vi "SetText.vi"(4 "Alignment":T1, 5 "Alpha":dbl=1.0, 7 "Color":u32(colorbox), 8 "error in (no error)":errorcluster, 9 "Font Path":path, 10 "Text":string, 11 "3D Object in":refnum<class "3D Object.lvclass">) -> (0 "error out":errorcluster, 3 "3D Object out":refnum<class "3D Object.lvclass">)   [LabVIEW 2015, in "3D Object.lvclass"]
uses:
  3D Object.lvclass
  <vilib>/Utility/miscctls.llb/LVSceneTextAlignment.ctl
  3D Object.lvclass/3D Object.ctl
  <vilib>/picture/3D Picture Control/NI_3D Picture Control.lvlib
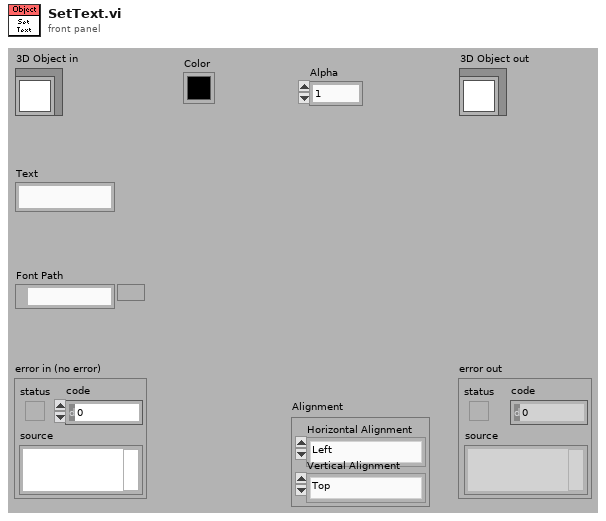
[diagram p1: front panel]
types:
  T1 = typedef "LVSceneTextAlignment.ctl" = cluster{"Horizontal Alignment":enum8{"Left", "Right", "Center"}, "Vertical Alignment":enum8{"Top", "Bottom", "Center", "Base Line", "Bottom Base Line"}}
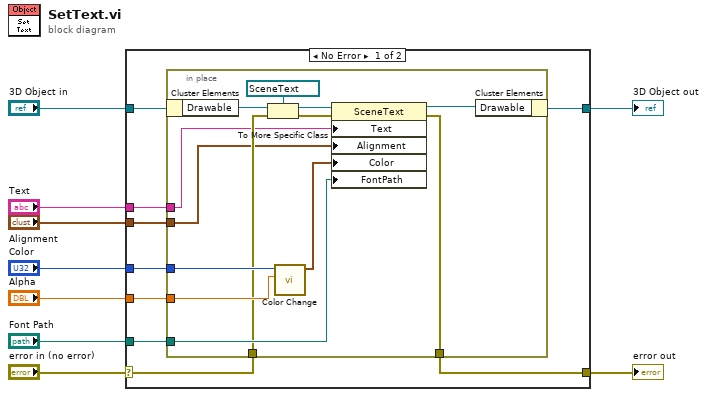
[diagram p0: block diagram]
diagram:
  n1 = case shown="No Error" "error in (no error)" {
    selector: "error in (no error)" -> [w12 w33]
    tunnel: [w17 w33] -> w8
    tunnel: [w10 w32] -> w6
    tunnel: "3D Object in" -> [w11 w32]
    tunnel: "Text" -> [w18 _]
    tunnel: "Font Path" -> [w14 _]
    tunnel: "Alignment" -> [w16 _]
    tunnel: "Color" -> [w15 _]
    tunnel: "Alpha" -> [w13 _]
    frame No Error {
      n2 = in-place {
        in-place-border: w18 -> [w19]
        in-place-border: [w31] -> w17
        in-place-border: w16 -> [w20]
        in-place-border: w15 -> [w30]
        in-place-border: w14 -> [w29]
        in-place-border: w13 -> [w28]
        in-place-border: w12 -> [w24]
        n3 = in-place-cluster #1(w11) -> ("Drawable"=w23:refnum<vi>)
        n4 = To More Specific Class(target class=refnum<vi> refnum ("reference"), reference=w23, error in=w24) -> (specific class reference=w25:refnum<vi>, error out=w27:errorcluster)
        n5 = call <vilib>:"Color Change.vi"("Alpha"=w28, "Color"=w30) -> ("RGBA"=w21:cluster{"R":sgl, "G":sgl, "B":sgl, "A":sgl})  [unwired: 9 out]
        n6 = property class="SceneText"(reference=w25, error in=w27, "Text"=w19, "Alignment"=w20, "Color"=w21, "FontPath"=w29) -> (reference out=w22:refnum<vi>, error out=w31:errorcluster)
        n7 = in-place-cluster #1("Drawable"=w22) -> (w10:refnum<class "3D Object.lvclass">)
      }
    }
    frame Error {
    }
  }
  "error out" <- w8
  "3D Object out" <- w6
